vi "main.vi"() -> ()   [LabVIEW 2021]
uses:
  FGVs/FGVstates.ctl
  <vilib>/Utility/inputDevices.llb/keyboardAcquire.vi
  <vilib>/Utility/inputDevices.llb/closeKeyboard.vi
panel:
  in  "Cancel Button":bool
  in  "error in (no error)":errorcluster
  out "error out":errorcluster
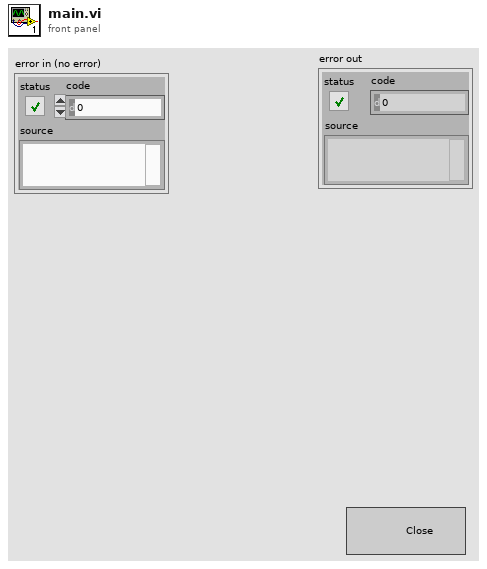
[diagram p1: front panel]
types:
  T1 = typedef "FGVstates.ctl" = enum16{"Init", "Set", "Get", "De-Init"}
  T2 = enum16{"0", "1", "2", "3", "4", "5", "6", "7", "8", "9", "A", "B", "C", "D", "E", "F", "G", "H", "I", "J", "K", "L", "M", "N", "O", "P", "Q", "R", "S", "T", "U", "V", "W", "X", "Y", "Z", "F1", "F2", "F3", "F4", "F5", "F6", "F7", "F8", "F9", "F10", "F11", "F12", "F13", "F14", "F15", "ADD", "BACK", "BACKSLASH", "CAPITAL", "COMMA", "DECIMAL", "DELETE", "DIVIDE", "DOWN", "END", "EQUALS", "ESCAPE", "GRAVE (`)", "HOME", "INSERT", "LBRACKET", "LCONTROL", "LEFT", "L ALT", "LSHIFT", "LWIN", "MINUS", "MULTIPLY", "NEXT", "NUMLOCK", "NUMPAD_0", "NUMPAD_1", "NUMPAD_2", "NUMPAD_3", "NUMPAD_4", "NUMPAD_5", "NUMPAD_6", "NUMPAD_7", "NUMPAD_8", "NUMPAD_9", "PAUSE", "PERIOD", "PRIOR (PG UP)", "RBRACKET", "RCONTROL", "RETURN", "RIGHT", "R ALT", "RSHIFT", "RWIN", "SCROLL", "SEMICOLON", "SLASH", "SPACE", "SUBTRACT", "TAB", "UP", "ENTER (num pad)", "' (quote)"}[]
  T3 = enum16{"0", "1", "2", "3", "4", "5", "6", "7", "8", "9", "A", "B", "C", "D", "E", "F", "G", "H", "I", "J", "K", "L", "M", "N", "O", "P", "Q", "R", "S", "T", "U", "V", "W", "X", "Y", "Z", "F1", "F2", "F3", "F4", "F5", "F6", "F7", "F8", "F9", "F10", "F11", "F12", "F13", "F14", "F15", "ADD", "BACK", "BACKSLASH", "CAPITAL", "COMMA", "DECIMAL", "DELETE", "DIVIDE", "DOWN", "END", "EQUALS", "ESCAPE", "GRAVE (`)", "HOME", "INSERT", "LBRACKET", "LCONTROL", "LEFT", "L ALT", "LSHIFT", "LWIN", "MINUS", "MULTIPLY", "NEXT", "NUMLOCK", "NUMPAD_0", "NUMPAD_1", "NUMPAD_2", "NUMPAD_3", "NUMPAD_4", "NUMPAD_5", "NUMPAD_6", "NUMPAD_7", "NUMPAD_8", "NUMPAD_9", "PAUSE", "PERIOD", "PRIOR (PG UP)", "RBRACKET", "RCONTROL", "RETURN", "RIGHT", "R ALT", "RSHIFT", "RWIN", "SCROLL", "SEMICOLON", "SLASH", "SPACE", "SUBTRACT", "TAB", "UP", "ENTER (num pad)", "' (quote)"}
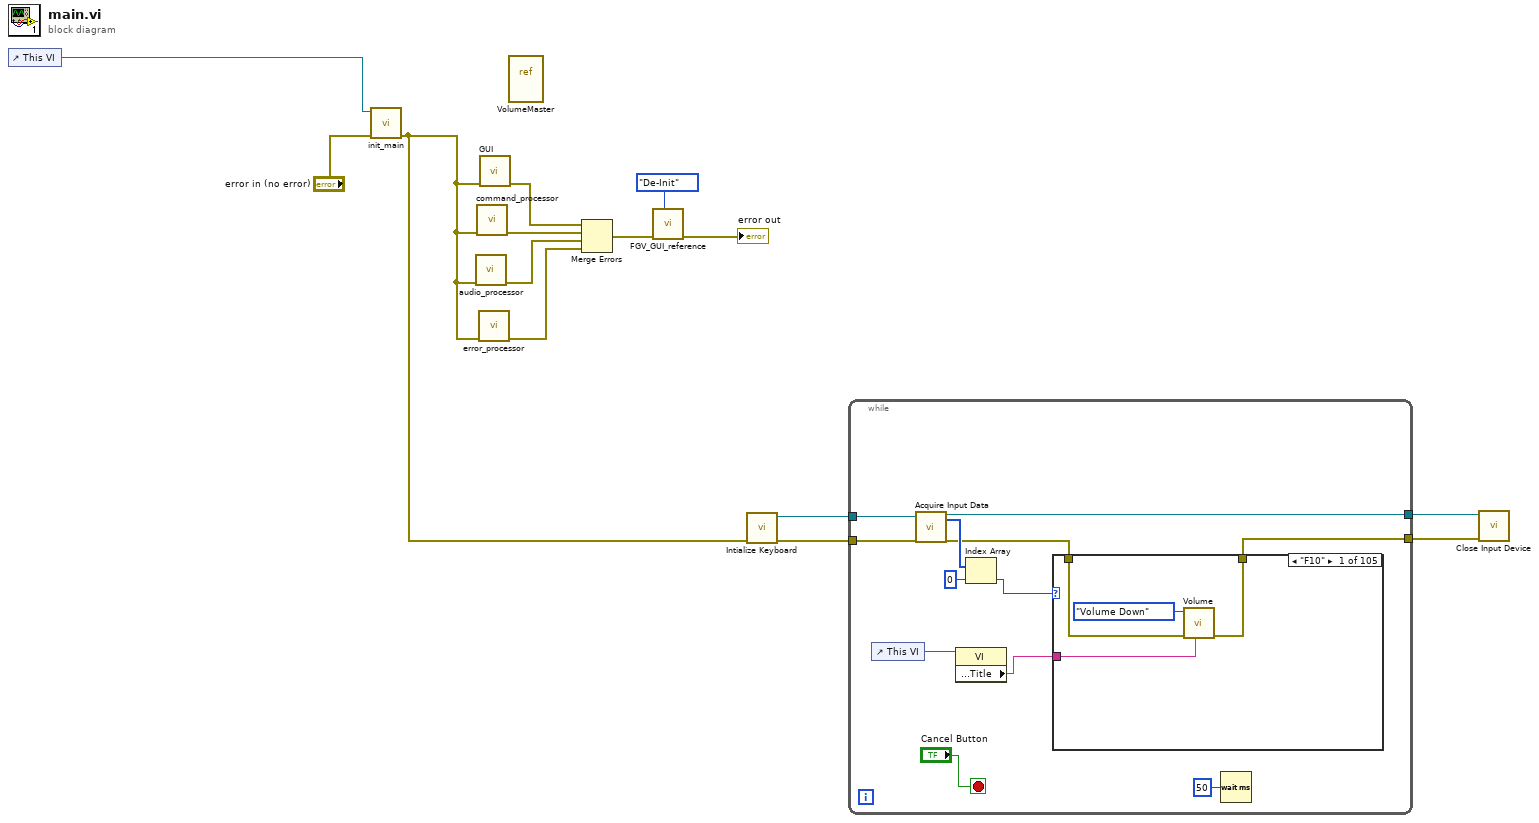
[diagram p0: block diagram]
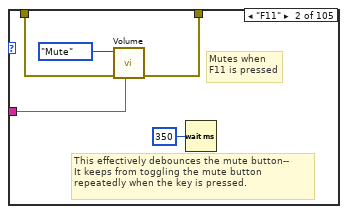
[diagram p2: hidden frame]
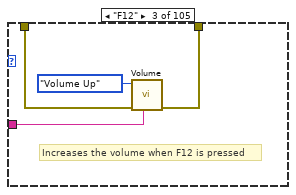
[diagram p3: hidden frame]
diagram:
  n1 = control-ref of="This VI"() -> (w10:refnum<vi>)
  n2 = call "init_main.vi"("error in (no error)"="error in (no error)", "VI in"=w10) -> ("error out"=w1:errorcluster)  [unwired: 9 in]
  n3 = call "audio_processor.vi"("error in (no error)"=w1) -> ("error out"=w12:errorcluster)  [unwired: 10 in]
  n4 = call "command_processor.vi"("error in (no error)"=w1) -> ("error out"=w13:errorcluster)  [unwired: 10 in]
  n5 = call "error_processor.vi"("error in (no error)"=w1) -> ("error out"=w11:errorcluster)  [unwired: 10 in]
  n6 = call "GUI.vi"("error in (no error)"=w1) -> ("error out"=w14:errorcluster)  [unwired: 10 in]
  n7 = vi-ref "VolumeMaster.vi"() -> ()  [unwired: 1 out]
  n8 = Merge Errors(w14, w13, w12, w11) -> (w7:errorcluster)
  n9 = call "FGV_GUI_reference.vi"("FGV states"=FGVstates."De-Init", "error in (no error)"=w7) -> ("error out"=→"error out":errorcluster)  [unwired: 8 in, 1 out]
  n10 = call <vilib>:"Intialize Keyboard.vi"("error in (no error)"=w1) -> ("error out"=w4:errorcluster, "device ID"=w5:refnum<k1>)  [unwired: 9 in]
  n11 = while {
    tunnel: w5 -> [w26]
    tunnel: w4 -> [w25]
    tunnel: [w21] -> w3
    tunnel: [w19] -> w2
    stop <- "Cancel Button" stop-if-true
    n12 = control-ref of="This VI"() -> (w16:refnum<vi>)
    n13 = call-poly <vilib>:"Acquire Input Data.vi"("device ID"=w26, "error in (no error)"=w25) -> ("device ID"=w21:refnum<k1>, "keys pressed"=w24:T2, "error out"=w20:errorcluster)  [unwired: 15 in]
    n14 = property class="VI"(reference=w16) -> ("Front Panel.Title"=w15:string)  [unwired: 1 in, 2 out]
    n15 = Index Array(array=w24, index=0) -> (element=w18:T3)
    n16 = case shown="\"F10\"" w18 {
      tunnel: w20 -> [w29 w34 w38 w40 w41 w42 w43 w44 w45 w46 w47 w48 w49 w50 w51 w52 w53 w54 w55 w56 w57 w58 w59 w60 w61 w62 w63 w64 w65 w66 w67 w68 w69 w70 w71 w72 w73 w74 w75 w76 w77 w78 w79 w80 w81 w82 w83 w84 w85 w86 w87 w88 w89 w90 w91 w92 w93 w94 w95 w96 w97 w98 w99 w100 w101 w102 w103 w104 w105 w106 w107 w108 w109 w110 w111 w112 w113 w114 w115 w116 w117 w118 w119 w120 w121 w122 w123 w124 w125 w126 w127 w128 w129 w130 w131 w132 w133 w134 w135 w136 w137 w138 w139 w140 w141]
      tunnel: [w28 w33 w37 w40 w41 w42 w43 w44 w45 w46 w47 w48 w49 w50 w51 w52 w53 w54 w55 w56 w57 w58 w59 w60 w61 w62 w63 w64 w65 w66 w67 w68 w69 w70 w71 w72 w73 w74 w75 w76 w77 w78 w79 w80 w81 w82 w83 w84 w85 w86 w87 w88 w89 w90 w91 w92 w93 w94 w95 w96 w97 w98 w99 w100 w101 w102 w103 w104 w105 w106 w107 w108 w109 w110 w111 w112 w113 w114 w115 w116 w117 w118 w119 w120 w121 w122 w123 w124 w125 w126 w127 w128 w129 w130 w131 w132 w133 w134 w135 w136 w137 w138 w139 w140 w141] -> w19
      tunnel: w15 -> [w27 w31 w36 _ _ _ _ _ _ _ _ _ _ _ _ _ _ _ _ _ _ _ _ _ _ _ _ _ _ _ _ _ _ _ _ _ _ _ _ _ _ _ _ _ _ _ _ _ _ _ _ _ _ _ _ _ _ _ _ _ _ _ _ _ _ _ _ _ _ _ _ _ _ _ _ _ _ _ _ _ _ _ _ _ _ _ _ _ _ _ _ _ _ _ _ _ _ _ _ _ _ _ _ _ _]
      frame "F10" {
        n17 = call "Volume.vi"("lpszWindowName"=w27, "error in (no error)"=w29, "Enum"=enum16{"Mute", "Volume Up", "Volume Down"}."Volume Down") -> ("error out"=w28:errorcluster)  [unwired: 8 in]
      }
      frame "F11" {
        # "Mutes when\nF11 is pressed"
        # "This effectively debounces the mute button--\nIt keeps from toggling the mute button\nrepeatedly when the key is pressed."
        n18 = call "Volume.vi"("lpszWindowName"=w31, "error in (no error)"=w34, "Enum"=enum16{"Mute", "Volume Up", "Volume Down"}."Mute") -> ("error out"=w33:errorcluster)  [unwired: 8 in]
        n19 = Wait (ms)(milliseconds to wait=u32 350) -> ()  [unwired: 1 out]
      }
      frame "F12" {
        # "Increases the volume when F12 is pressed"
        n20 = call "Volume.vi"("lpszWindowName"=w36, "error in (no error)"=w38, "Enum"=enum16{"Mute", "Volume Up", "Volume Down"}."Volume Up") -> ("error out"=w37:errorcluster)  [unwired: 8 in]
      }
      frame "F13" {
      }
      frame "F14" {
      }
      frame "F15" {
      }
      frame "ADD" {
      }
      frame "BACK" {
      }
      frame "BACKSLASH" {
      }
      frame "CAPITAL" {
      }
      frame "COMMA" {
      }
      frame "DECIMAL" {
      }
      frame "DELETE" {
      }
      frame "DIVIDE" {
      }
      frame "DOWN" {
      }
      frame "END" {
      }
      frame "EQUALS" {
      }
      frame "ESCAPE" {
      }
      frame "GRAVE (`)" {
      }
      frame "HOME" {
      }
      frame "INSERT" {
      }
      frame "LBRACKET" {
      }
      frame "LCONTROL" {
      }
      frame "LEFT" {
      }
      frame "L ALT" {
      }
      frame "LSHIFT" {
      }
      frame "LWIN" {
      }
      frame "MINUS" {
      }
      frame "MULTIPLY" {
      }
      frame "NEXT" {
      }
      frame "NUMLOCK" {
      }
      frame "NUMPAD_0" {
      }
      frame "NUMPAD_1" {
      }
      frame "NUMPAD_2" {
      }
      frame "NUMPAD_3" {
      }
      frame "NUMPAD_4" {
      }
      frame "NUMPAD_5" {
      }
      frame "NUMPAD_6" {
      }
      frame "NUMPAD_7" {
      }
      frame "NUMPAD_8" {
      }
      frame "NUMPAD_9" {
      }
      frame "PAUSE" {
      }
      frame "PERIOD" {
      }
      frame "PRIOR (PG UP)" {
      }
      frame "RBRACKET" {
      }
      frame "RCONTROL" {
      }
      frame "RETURN" {
      }
      frame "RIGHT" {
      }
      frame "R ALT" {
      }
      frame "RSHIFT" {
      }
      frame "RWIN" {
      }
      frame "SCROLL" {
      }
      frame "SEMICOLON" {
      }
      frame "SLASH" {
      }
      frame "SPACE" {
      }
      frame "SUBTRACT" {
      }
      frame "TAB" {
      }
      frame "UP" {
      }
      frame "ENTER (num pad)" {
      }
      frame "' (quote)" {
      }
      frame "F9" {
      }
      frame "F8" {
      }
      frame "F7" {
      }
      frame "F6" {
      }
      frame "F5" {
      }
      frame "F4" {
      }
      frame "F3" {
      }
      frame "F2" {
      }
      frame "F1" {
      }
      frame "Z" {
      }
      frame "Y" {
      }
      frame "X" {
      }
      frame "W" {
      }
      frame "V" {
      }
      frame "U" {
      }
      frame "T" {
      }
      frame "S" {
      }
      frame "R" {
      }
      frame "Q" {
      }
      frame "P" {
      }
      frame "O" {
      }
      frame "N" {
      }
      frame "M" {
      }
      frame "L" {
      }
      frame "K" {
      }
      frame "J" {
      }
      frame "I" {
      }
      frame "H" {
      }
      frame "G" {
      }
      frame "F" {
      }
      frame "E" {
      }
      frame "D" {
      }
      frame "C" {
      }
      frame "B" {
      }
      frame "A" {
      }
      frame "9" {
      }
      frame "8" {
      }
      frame "7" {
      }
      frame "6" {
      }
      frame "5" {
      }
      frame "4" {
      }
      frame "3" {
      }
      frame "2" {
      }
      frame "1" {
      }
      frame "0" {
      }
    }
    n21 = Wait (ms)(milliseconds to wait=u32 50) -> ()  [unwired: 1 out]
  }
  n22 = call-poly <vilib>:"Close Input Device.vi"("error in (no error)"=w2, "device ID"=w3) -> ()  [unwired: 8 in, 1 out]
